vi "Start Framegrabber.vi"(1 "Cluster In":T3, 2 "Enable?":bool, 3 "Bool Refnum":refnum<vi>) -> (0 "Cluster Out":T3)   [LabVIEW 2010]
uses:
  System.Windows.Forms
  drivers/DirectShow SDK/v10/DirectShow SDK.llb/DirectShow - Capture Device.ctl
  D:/Projekte/Promotion/Scripts/LabView/drivers/DirectShow SDK/lib/DirectShowLib-2005.dll
  drivers/DirectShow SDK/lib/DirectShowLib-2005.dll
  drivers/DirectShow SDK/v10/DirectShow SDK.llb/DirectShow - Media State.ctl
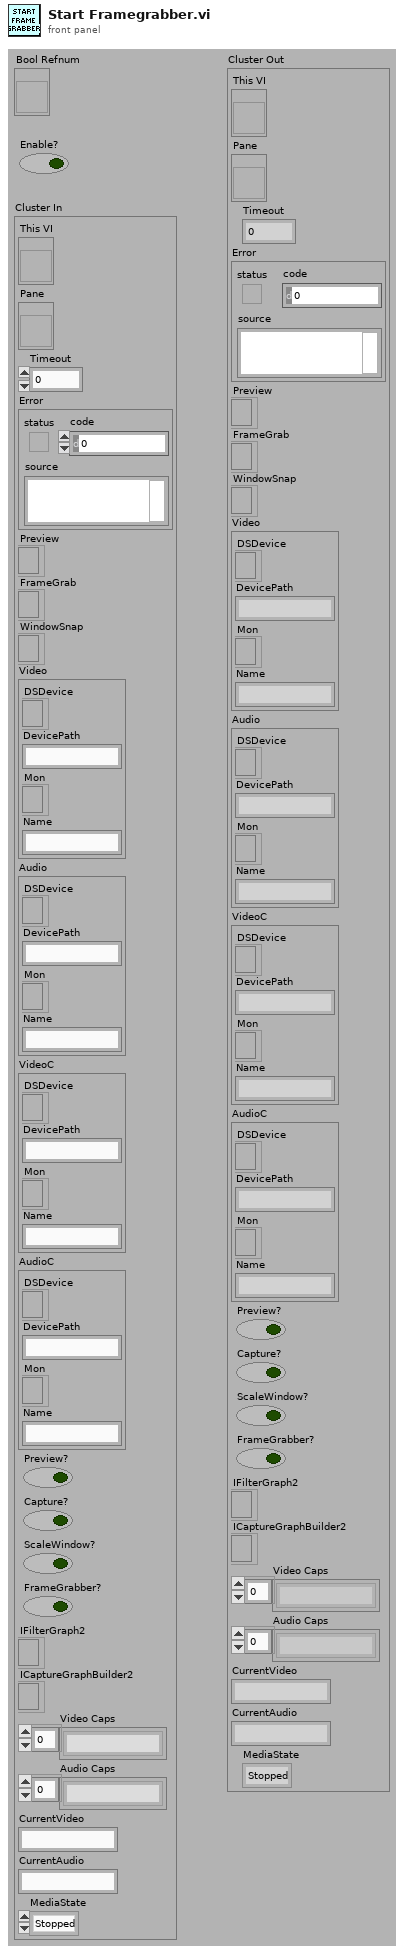
[diagram p1: front panel]
types:
  T1 = typedef "DirectShow - Capture Device.ctl" = cluster{"DSDevice":refnum<k24>, "DevicePath":string, "Mon":refnum<k24>, "Name":string}
  T2 = typedef "DirectShow - Media State.ctl" = enum16{"Stopped", "Playing", "Paused", "Recording"}
  T3 = cluster{"This VI":refnum<vi>, "Pane":refnum<vi>, "Timeout":i32, "Error":errorcluster, "Preview":refnum<k24>, "FrameGrab":refnum<k24>, "WindowSnap":refnum<k24>, "Video":T1, "Audio":T1, "VideoC":T1, "AudioC":T1, "Preview?":bool, "Capture?":bool, "ScaleWindow?":bool, "FrameGrabber?":bool, "IFilterGraph2":refnum<k24>, "ICaptureGraphBuilder2":refnum<k24>, "Video Caps":string[], "Audio Caps":string[], "CurrentVideo":string, "CurrentAudio":string, "MediaState":T2}
  T4 = enum8{"Enabled", "Disabled", "Disabled and Grayed Out"}
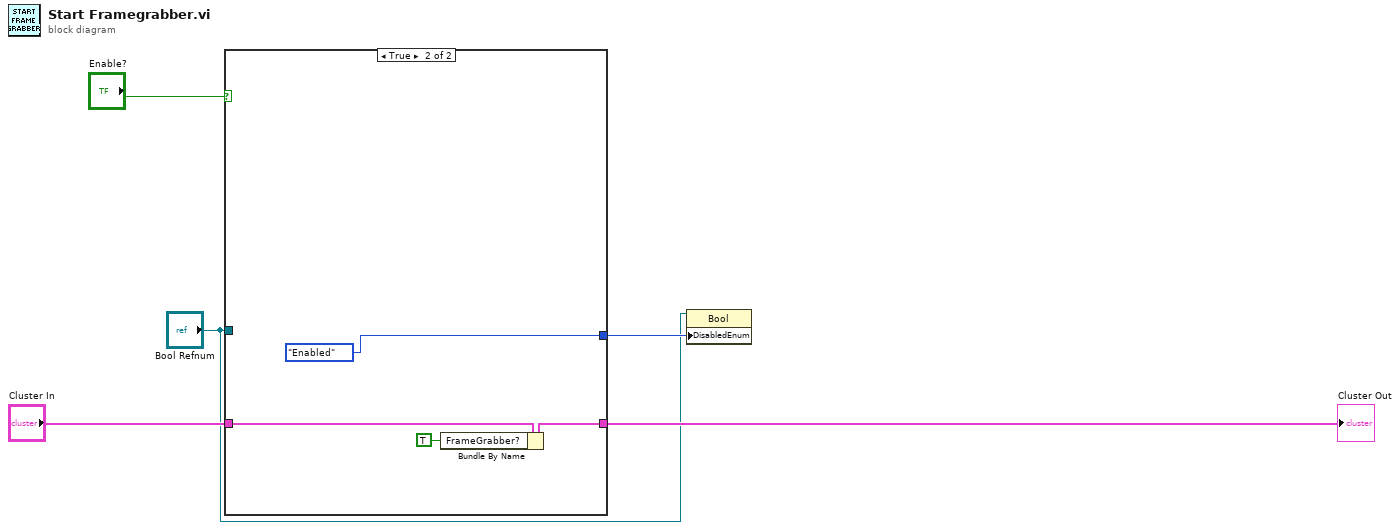
[diagram p0: block diagram]
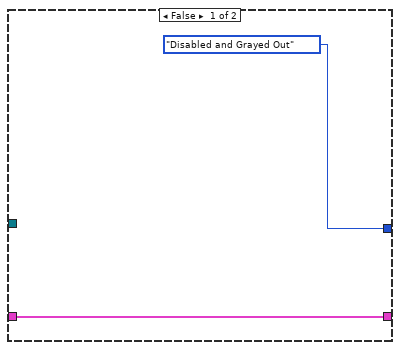
[diagram p2: hidden frame]
diagram:
  n1 = case shown="True" "Enable?" {
    tunnel: "Cluster In" -> [w7 w11]
    tunnel: [w7 w10] -> w4
    tunnel: "Bool Refnum" -> [_ _]
    tunnel: [T4."Disabled and Grayed Out" ("Disabled") T4."Enabled" ("Disabled")] -> w2
    frame False {
    }
    frame True {
      n2 = Bundle By Name(cluster=w11, "FrameGrabber?"=TRUE) -> (w10:T3)
    }
  }
  "Cluster Out" <- w4
  n3 = property on="Property Node" class="Bool"(reference="Bool Refnum", "DisabledEnum"=w2) -> ()  [unwired: 1 in, 2 out]
